vi "DAQmx连续输出数量波形数据.vi"() -> ()   [LabVIEW 2010]
uses:
  <vilib>/DAQmx/write.llb/DAQmx Write.vi
  <vilib>/DAQmx/write.llb/DAQmx Write (Analog 1D Wfm NChan NSamp).vi
  <vilib>/daqmx/miscellaneous.llb/DAQmx Fill In Error Info.vi
  <vilib>/measure/NI_MABase.lvlib
panel:
  in  "stop":bool
  in  "amplitude":dbl=1.0 format="%0.2p"
  in  "frequency":dbl=10.0 format="%0.2p"
  in  "signal type":T1(ring)
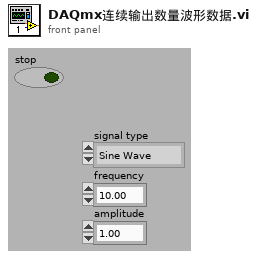
[diagram p1: front panel]
types:
  T1 = enum16{"Sine Wave", "Triangle Wave", "Square Wave", "Sawtooth Wave"}
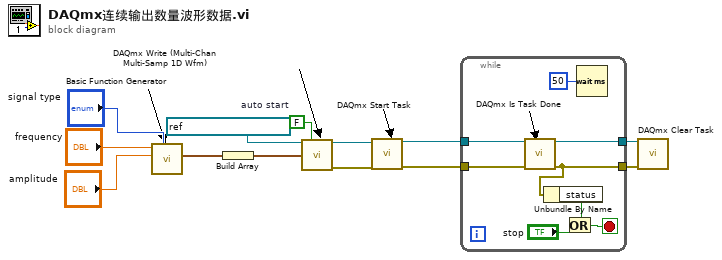
[diagram p0: block diagram]
diagram:
  w13 = FALSE  # auto start
  n1 = call <vilib>:"Basic Function Generator.vi"("signal type"="signal type", "amplitude"="amplitude", "frequency"="frequency") -> ("signal out"=w9:waveform(dbl))  [unwired: 6 in, 2 out]
  n2 = Build Array(w9) -> (w8:waveform(dbl)[])
  n3 = call-poly "DAQmx Write (Multi-Chan Multi-Samp 1D Wfm).vi"("task/channels in"=refnum<k21> "我的电压输出任务", "auto start"=w13, "data"=w8) -> ("task out"=w12:refnum<k21>, "error out"=w11:errorcluster)  [unwired: 10 in, 1 out]
  n4 = call <vilib>:"DAQmx Start Task.vi"("task/channels in"=w12, "error in"=w11) -> ("task out"=w4:refnum<k21>, "error out"=w2:errorcluster)  [unwired: 12 in]
  n5 = while {
    tunnel: w4 -> [w21]
    tunnel: [w20] -> w3
    tunnel: w2 -> [w19]
    tunnel: [w18] -> w1
    stop <- w17 stop-if-true
    n6 = call <vilib>:"DAQmx Is Task Done.vi"("task/channels in"=w21, "error in"=w19) -> ("task out"=w20:refnum<k21>, "error out"=w18:errorcluster)  [unwired: 11 in, 1 out]
    n7 = Unbundle By Name(w18) -> ("status"=w16:bool)
    n8 = Or(x=w16, y="stop") -> (x .or. y?=w17:bool)
    n9 = Wait (ms)(milliseconds to wait=u32 50 ("等待时间（毫秒）")) -> ()  [unwired: 1 out]
  }
  n10 = call <vilib>:"DAQmx Clear Task.vi"("task in"=w3, "error in"=w1) -> ()  [unwired: 13 in, 1 out]
